vi "VI principal ( LES CHIFFRES ROMAINS).vi"() -> ()   [LabVIEW 2023]
panel:
  out "Numeric 3":dbl
  in  "ENTER AN ARAB NUMBER?":dbl
  in  "ok du roman number":bool
  out "?":string="entrez un nombre inferieur ou egale a 3000"
  out "ROMAIN NUMBER:":string
  in  "Cancel Button":bool
  in  "STOP Programme":bool
  in  "New conversion":bool
  in  "selection confirmed":bool
  in  "Enter a ROMAN  number?":string
  in  "ROMAN TO ARAB NUMBERS":string(combo) caption="WHICH CONVERSION YOU WANT?"
  in  "Arabic number":bool
  out "?":string="entrez un nombre inferieur ou egale a 3000"
  out "Arabic number:":dbl
  in  "Login":bool
  out "Login&Password":bool
  in  "Name":string
  in  "Password":string
  in  "First Name":string
  out "Message":string
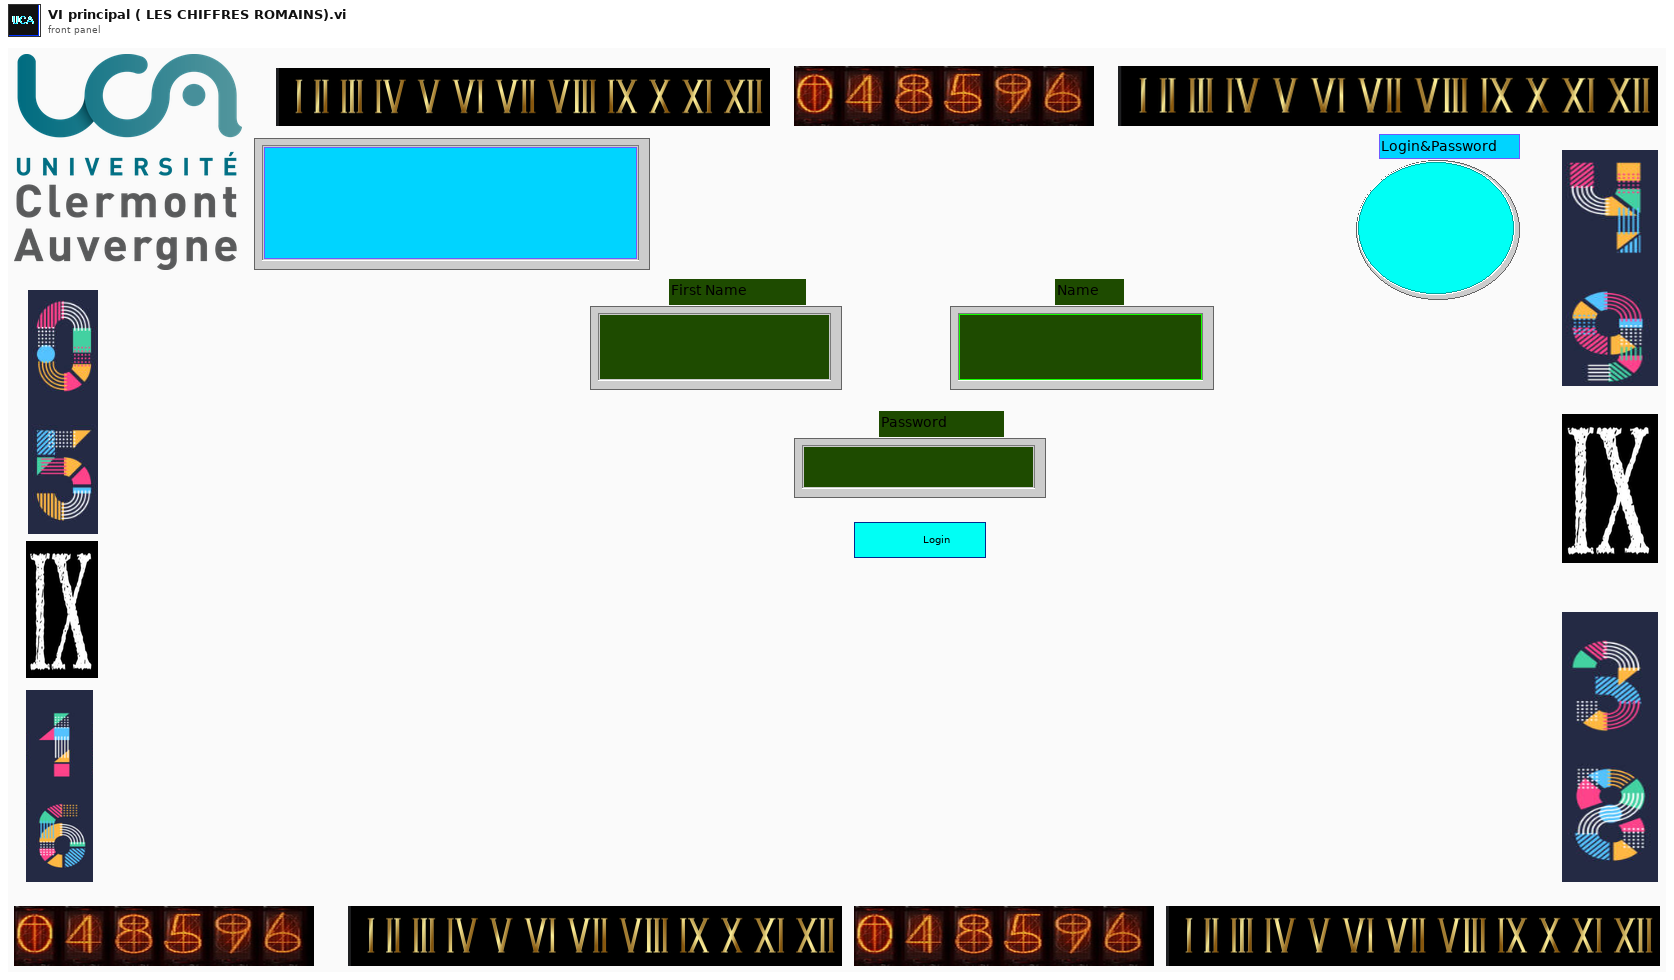
[diagram p1: front panel]
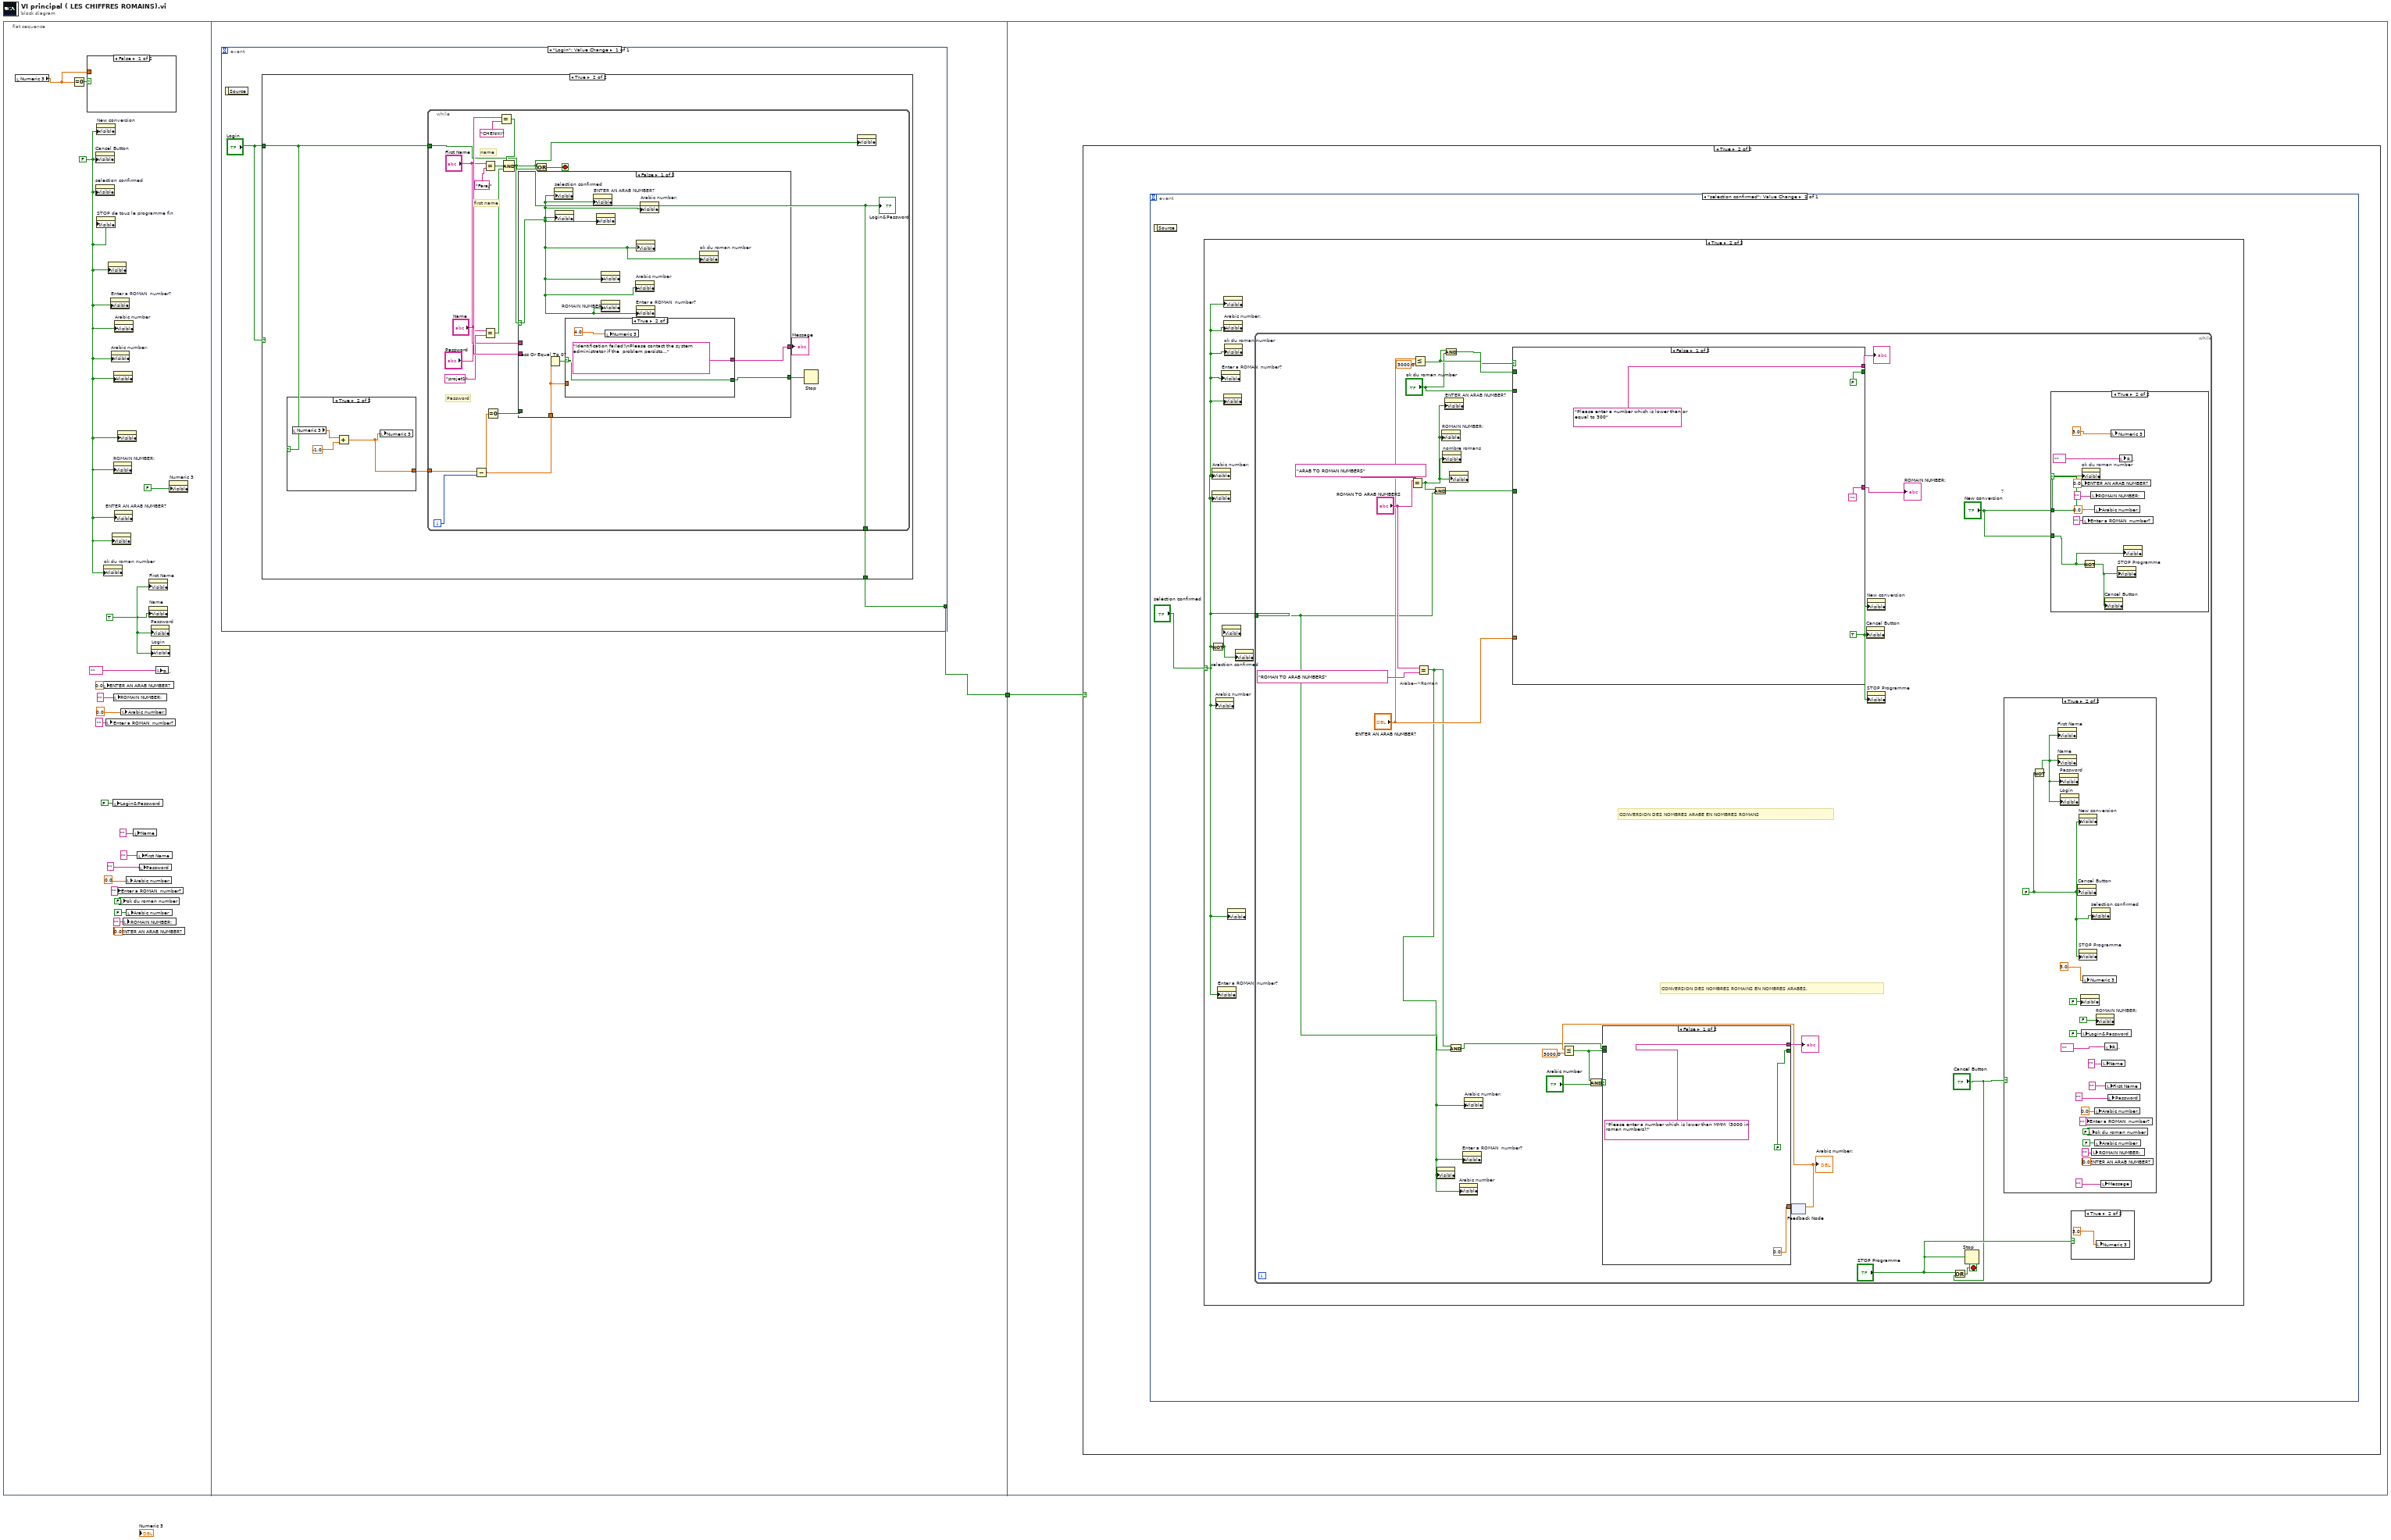
[diagram p0: block diagram]
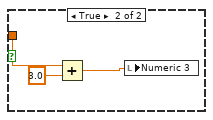
[diagram p2: hidden frame]
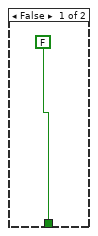
[diagram p3: hidden frame]
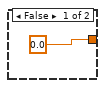
[diagram p4: hidden frame]
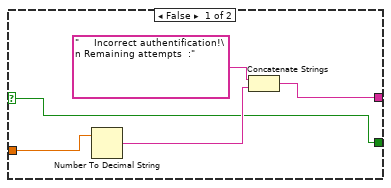
[diagram p5: hidden frame]
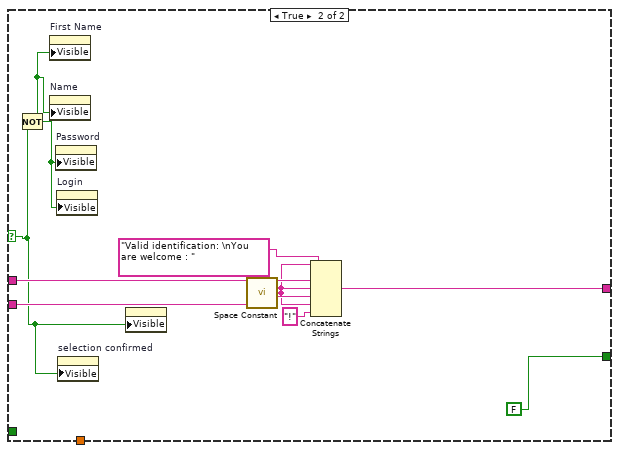
[diagram p6: hidden frame]
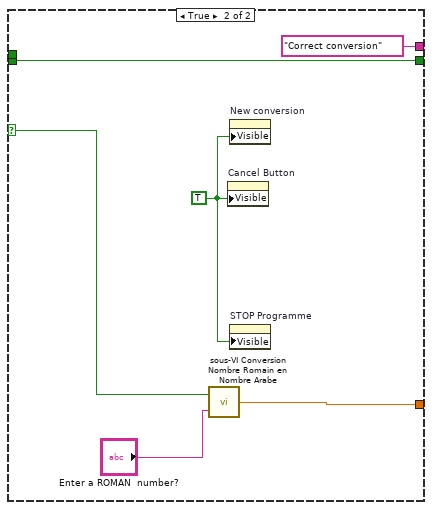
[diagram p12: hidden frame]
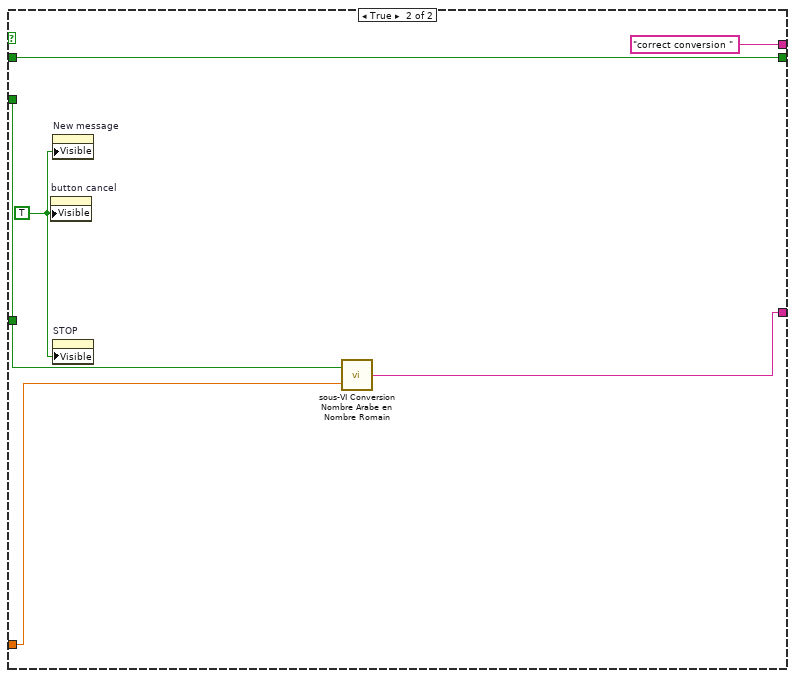
[diagram p13: hidden frame]
diagram:
  n1 = flat-sequence {
    tunnel: [w25] -> w1
    tunnel: w1 -> [w76]
    frame #0 {
      w5 = TRUE
      w21 = FALSE
      n2 = local read "Numeric 3"() -> (w2:dbl)
      n3 = Equal To 0?(x=w2) -> (x = 0?=w3:bool)
      n4 = case shown="False" w3 {
        tunnel: w2 -> [_ w24]
        frame False {
        }
        frame True {
          n5 = Add(x=w24, y=3.0) -> (x+y=w22:dbl)
          n6 = local write "Numeric 3"(w22) -> ()
        }
      }
      n7 = property on="Cancel Button" class="Bool"("Visible"=w21) -> ()  [unwired: 2 in, 2 out]
      n8 = property on="selection confirmed" class="Bool (strict)"("Visible"=w21) -> ()  [unwired: 2 in, 2 out]
      n9 = property on="New conversion" class="Bool"("Visible"=w21) -> ()  [unwired: 2 in, 2 out]
      n10 = property on="STOP de tous le programme fin" class="Bool"("Visible"=w21) -> ()  [unwired: 2 in, 2 out]
      n11 = local write "ENTER AN ARAB NUMBER?"(0.0 ("Nombre Arabe")) -> ()
      n12 = property on="ok du roman number" class="Bool (strict)"("Visible"=w21) -> ()  [unwired: 2 in, 2 out]
      n13 = local write "Enter a ROMAN  number?"("" ("Nombre romain 1")) -> ()
      n14 = property class="CmbBox"("Visible"=w21) -> ()  [unwired: 2 in, 2 out]
      n15 = property on="Enter a ROMAN  number?" class="Str"("Visible"=w21) -> ()  [unwired: 2 in, 2 out]
      n16 = property on="Arabic number:" class="DigNum (strict)"("Visible"=w21) -> ()  [unwired: 2 in, 2 out]
      n17 = property class="Str"("Visible"=w21) -> ()  [unwired: 2 in, 2 out]
      n18 = local write "Login&Password"(FALSE ("Login&Password")) -> ()
      n19 = property on="ROMAIN NUMBER:" class="Str"("Visible"=w21) -> ()  [unwired: 2 in, 2 out]
      n20 = local write "ROMAIN NUMBER:"("" ("Nombre Romain")) -> ()
      n21 = property class="CmbBox"("Visible"=w21) -> ()  [unwired: 2 in, 2 out]
      n22 = local write "Enter a ROMAN  number?"("" ("Nombre romain 1")) -> ()
      n23 = local write "ENTER AN ARAB NUMBER?"(0.0 ("Nombre Arabe")) -> ()
      n24 = property on="ENTER AN ARAB NUMBER?" class="DigNum (strict)"("Visible"=w21) -> ()  [unwired: 2 in, 2 out]
      n25 = property on="Arabic number" class="Bool (strict)"("Visible"=w21) -> ()  [unwired: 2 in, 2 out]
      n26 = property class="Str"("Visible"=w21) -> ()  [unwired: 2 in, 2 out]
      n27 = local write "ok du roman number"(FALSE ("Roman number")) -> ()
      n28 = local write "Arabic number:"(0.0 ("Nombre arabe 1")) -> ()
      n29 = local write "ROMAIN NUMBER:"("" ("Nombre Romain")) -> ()
      n30 = local write "Arabic number:"(0.0 ("Nombre arabe 1")) -> ()
      n31 = local write "Arabic number"(FALSE ("Arabic number")) -> ()
      n32 = local write "Name"("" ("First name:")) -> ()
      n33 = local write "First Name"("" ("Name:")) -> ()
      n34 = local write "Password"("" ("Password:")) -> ()
      n35 = property on="First Name" class="Str"("Visible"=w5) -> ()  [unwired: 2 in, 2 out]
      n36 = property on="Name" class="Str"("Visible"=w5) -> ()  [unwired: 2 in, 2 out]
      n37 = property on="Password" class="Str"("Visible"=w5) -> ()  [unwired: 2 in, 2 out]
      n38 = property on="Login" class="Bool (strict)"("Visible"=w5) -> ()  [unwired: 2 in, 2 out]
      n39 = local write "ROMAN TO ARAB NUMBERS"("" ("Choose your conversion")) -> ()
      n40 = property on="Numeric 3" class="DigNum (strict)"("Visible"=FALSE) -> ()  [unwired: 2 in, 2 out]
    }
    frame #1 {
      n41 = event shown="[0] \"Login\": Value Change" {
        selector: _ -> [_]
        dyn-events: _ -> [_]
        timeout: _ -> [_]
        tunnel: [w27] -> w25
        event "Login": Value Change {
          n42 = event-data() -> ()  [unwired: 1 in, 1 out]
          n43 = case shown="True" "Login" {
            tunnel: "Login" -> [_ w29]
            tunnel: [FALSE w31] -> w27
            frame False {
            }
            frame True {
              n44 = case shown="True" w29 {
                tunnel: [0.0 w33] -> w30
                frame False {
                }
                frame True {
                  n45 = local read "Numeric 3"() -> (w34:dbl)
                  n46 = Add(x=w34, y=-1.0) -> (x+y=w33:dbl)
                  n47 = local write "Numeric 3"(w33) -> ()
                }
              }
              n48 = while {
                tunnel: w29 -> [w39]
                tunnel: [w37] -> w31
                tunnel: w30 -> [w38]
                i -> [w40]
                stop <- w43 stop-if-true
                # "Password"
                # "first name"
                # "name"
                n49 = Subtract(x=w38, y=w40) -> (x-y=w41:dbl)
                n50 = Equal?(x="First Name", y="Faraj") -> (x = y?=w49:bool)
                n51 = Equal?(x="Password", y="projet1") -> (x = y?=w50:bool)
                n52 = Equal To 0?(x=w41) -> (x = 0?=w42:bool)
                n53 = Equal?(x="Name", y="CHENIKI") -> (x = y?=w48:bool)
                n54 = Compound Arithmetic op=AND(w48, w49, w50) -> (w37:bool)
                "Login&Password" <- w37
                n55 = case shown="False" w37 {
                  selector: w37 -> [w55 w68]
                  tunnel: [w57 w70] -> w53
                  tunnel: "First Name" -> [_ w74]
                  tunnel: "Name" -> [_ w73]
                  tunnel: w42 -> [_ _]
                  tunnel: w41 -> [w56 _]
                  tunnel: [w54 FALSE] -> w36
                  frame False {
                    n56 = Less Or Equal To 0?(x=w56) -> (x <= 0?=w58:bool)
                    n57 = property on="selection confirmed" class="Bool (strict)"("Visible"=w55) -> ()  [unwired: 2 in, 2 out]
                    n58 = property class="CmbBox"("Visible"=w55) -> ()  [unwired: 2 in, 2 out]
                    n59 = case shown="True" w58 {
                      selector: w58 -> [w59 w64]
                      tunnel: [w62 "Identification failed!\nPlease contact the system administrator if the  problem persists..." ("string")] -> w57
                      tunnel: w56 -> [w61 _]
                      tunnel: [w59 w64] -> w54
                      frame False {
                        n60 = Number To Decimal String(number=w61) -> (decimal integer string=w60:string)  [unwired: 1 in]
                        n61 = Concatenate Strings("     Incorrect authentification!\n Remaining attempts  :", w60) -> (w62:string)
                      }
                      frame True {
                        n62 = local write "Numeric 3"(4.0) -> ()
                      }
                    }
                    n63 = property on="ENTER AN ARAB NUMBER?" class="DigNum (strict)"("Visible"=w55) -> ()  [unwired: 2 in, 2 out]
                    n64 = property class="Str"("Visible"=w55) -> ()  [unwired: 2 in, 2 out]
                    n65 = property class="Str"("Visible"=w55) -> ()  [unwired: 2 in, 2 out]
                    n66 = property on="ROMAIN NUMBER:" class="Str"("Visible"=w55) -> ()  [unwired: 2 in, 2 out]
                    n67 = property on="Arabic number" class="Bool (strict)"("Visible"=w55) -> ()  [unwired: 2 in, 2 out]
                    n68 = property on="Enter a ROMAN  number?" class="Str"("Visible"=w55) -> ()  [unwired: 2 in, 2 out]
                    n69 = property class="Str"("Visible"=w55) -> ()  [unwired: 2 in, 2 out]
                    n70 = property on="Arabic number:" class="DigNum (strict)"("Visible"=w55) -> ()  [unwired: 2 in, 2 out]
                    n71 = property on="ok du roman number" class="Bool (strict)"("Visible"=w55) -> ()  [unwired: 2 in, 2 out]
                  }
                  frame True {
                    n72 = Not(x=w68) -> (.not. x?=w69:bool)
                    n73 = property on="First Name" class="Str"("Visible"=w69) -> ()  [unwired: 2 in, 2 out]
                    n74 = property on="Name" class="Str"("Visible"=w69) -> ()  [unwired: 2 in, 2 out]
                    n75 = property on="Password" class="Str"("Visible"=w69) -> ()  [unwired: 2 in, 2 out]
                    n76 = property on="Login" class="Bool (strict)"("Visible"=w69) -> ()  [unwired: 2 in, 2 out]
                    n77 = property on="selection confirmed" class="Bool (strict)"("Visible"=w68) -> ()  [unwired: 2 in, 2 out]
                    n78 = property class="CmbBox"("Visible"=w68) -> ()  [unwired: 2 in, 2 out]
                    n79 = call <vilib>:"Space Constant.vi"() -> ("String"=w72:string)
                    n80 = Concatenate Strings("Valid identification: \nYou are welcome : ", w72, w74, w72, w73, w72, "!") -> (w70:string)
                  }
                }
                "Message" <- w53
                n81 = Or(x=w37, y=w39) -> (x .or. y?=w43:bool)
                n82 = Stop(stop? (T)=w36) -> ()
                n83 = property class="CmbBox"("Visible"=w37) -> ()  [unwired: 2 in, 2 out]
              }
            }
          }
        }
      }
    }
    frame #2 {
      n84 = case shown="True" w76 {
        frame False {
        }
        frame True {
          n85 = event shown="[0] \"selection confirmed\": Value Change" {
            selector: _ -> [_]
            dyn-events: _ -> [_]
            timeout: _ -> [_]
            event "selection confirmed": Value Change {
              n86 = event-data() -> ()  [unwired: 1 in, 1 out]
              n87 = case shown="True" "selection confirmed" {
                selector: "selection confirmed" -> [_ w79]
                frame False {
                }
                frame True {
                  n88 = Not(x=w79) -> (.not. x?=w78:bool)
                  n89 = property on="Arabic number:" class="DigNum (strict)"("Visible"=w79) -> ()  [unwired: 2 in, 2 out]
                  n90 = property class="Str"("Visible"=w79) -> ()  [unwired: 2 in, 2 out]
                  n91 = property on="Arabic number" class="Bool (strict)"("Visible"=w79) -> ()  [unwired: 2 in, 2 out]
                  n92 = property on="Enter a ROMAN  number?" class="Str"("Visible"=w79) -> ()  [unwired: 2 in, 2 out]
                  n93 = property on="Enter a ROMAN  number?" class="Str"("Visible"=w79) -> ()  [unwired: 2 in, 2 out]
                  n94 = property class="CmbBox"("Visible"=w78) -> ()  [unwired: 2 in, 2 out]
                  n95 = property class="Str"("Visible"=w79) -> ()  [unwired: 2 in, 2 out]
                  n96 = property class="CmbBox"("Visible"=w79) -> ()  [unwired: 2 in, 2 out]
                  n97 = property on="Arabic number:" class="DigNum (strict)"("Visible"=w79) -> ()  [unwired: 2 in, 2 out]
                  n98 = property on="ok du roman number" class="Bool (strict)"("Visible"=w79) -> ()  [unwired: 2 in, 2 out]
                  n99 = property class="Str"("Visible"=w79) -> ()  [unwired: 2 in, 2 out]
                  n100 = property on="selection confirmed" class="Bool (strict)"("Visible"=w78) -> ()  [unwired: 2 in, 2 out]
                  n101 = while {
                    tunnel: w79 -> [w91]
                    stop <- w87 stop-if-true
                    w90 = TRUE
                    # "CONVERSION DES NOMBRES ARABE EN NOMBRES ROMANS"
                    # "CONVERSION DES NOMBRES ROMAINS EN NOMBRES ARABES."
                    # "?"
                    # "Arabe-->Roman"
                    n102 = Equal?(x="ROMAN TO ARAB NUMBERS", y="ARAB TO ROMAN NUMBERS") -> (x = y?=w96:bool)
                    n103 = Less Or Equal?(x="ENTER AN ARAB NUMBER?", y=3000.0) -> (x <= y?=w100:bool)
                    n104 = Equal?(x="ROMAN TO ARAB NUMBERS", y="ROMAN TO ARAB NUMBERS") -> (x = y?=w80:bool)
                    n105 = And(x=w96, y=w91) -> (x .and. y?=w97:bool)
                    n106 = property class="Str"("Visible"=w80) -> ()  [unwired: 2 in, 2 out]
                    n107 = property on="ROMAIN NUMBER:" class="Str"("Visible"=w96) -> ()  [unwired: 2 in, 2 out]
                    n108 = property on="nombre romans" class="Bool (strict)"("Visible"=w96) -> ()  [unwired: 2 in, 2 out]
                    n109 = And(x=w100, y="ok du roman number") -> (x .and. y?=w98:bool)
                    n110 = property on="ENTER AN ARAB NUMBER?" class="DigNum (strict)"("Visible"=w96) -> ()  [unwired: 2 in, 2 out]
                    n111 = And(x=w80, y=w91) -> (x .and. y?=w81:bool)
                    n112 = property class="Str"("Visible"=w96) -> ()  [unwired: 2 in, 2 out]
                    n113 = property on="Arabic number" class="Bool (strict)"("Visible"=w80) -> ()  [unwired: 2 in, 2 out]
                    n114 = property on="Enter a ROMAN  number?" class="Str"("Visible"=w80) -> ()  [unwired: 2 in, 2 out]
                    n115 = property on="Arabic number:" class="DigNum (strict)"("Visible"=w80) -> ()  [unwired: 2 in, 2 out]
                    n116 = case shown="False" w98 {
                      tunnel: "ENTER AN ARAB NUMBER?" -> [_ w148]
                      tunnel: ["Please enter a number which is lower than or equal to 300" "correct conversion "] -> w101
                      tunnel: w100 -> [_ w151]
                      tunnel: [FALSE w151] -> _
                      tunnel: ["" w147] -> w99
                      tunnel: w97 -> [_ _]
                      tunnel: "ok du roman number" -> [_ w146]
                      frame False {
                      }
                      frame True {
                        w149 = TRUE
                        n117 = property on="button cancel" class="Bool"("Visible"=w149) -> ()  [unwired: 2 in, 2 out]
                        n118 = property on="New message" class="Bool"("Visible"=w149) -> ()  [unwired: 2 in, 2 out]
                        n119 = property on="STOP" class="Bool"("Visible"=w149) -> ()  [unwired: 2 in, 2 out]
                        n120 = call "sous-VI Conversion Nombre Arabe en Nombre Romain.vi"("Enter AN ARABIC NUMBER?"=w148, "Roman number"=w146) -> ("ROMAN NUMBER:"=w147:string)
                      }
                    }
                    "?" <- w101
                    "ROMAIN NUMBER:" <- w99
                    n121 = feedback #1() -> (w85:dbl)  [unwired: 1 in]
                    "Arabic number:" <- w85
                    n122 = Less Or Equal?(x=w85, y=3000.0) -> (x <= y?=w95:bool)
                    n123 = And(x=w95, y="Arabic number") -> (x .and. y?=w92:bool)
                    n124 = case shown="False" w92 {
                      selector: w92 -> [_ w138]
                      tunnel: ["Please enter a number which is lower than MMM  (3000 in roman numbers)!" "Correct conversion"] -> w94
                      tunnel: [FALSE w141] -> _
                      tunnel: w95 -> [_ w141]
                      tunnel: [0.0 w139] -> w86
                      tunnel: w81 -> [_ _]
                      frame False {
                      }
                      frame True {
                        w140 = TRUE
                        n125 = call "sous-VI Conversion Nombre Romain en Nombre Arabe.vi"("Enter a ROMAN nomber?"="Enter a ROMAN  number?", "RESULT"=w138) -> ("Arabic number:"=w139:dbl)
                        n126 = property on="Cancel Button" class="Bool"("Visible"=w140) -> ()  [unwired: 2 in, 2 out]
                        n127 = property on="New conversion" class="Bool"("Visible"=w140) -> ()  [unwired: 2 in, 2 out]
                        n128 = property on="STOP Programme" class="Bool"("Visible"=w140) -> ()  [unwired: 2 in, 2 out]
                      }
                    }
                    "?" <- w94
                    n129 = feedback-in #1(w86) -> ()
                    n130 = property on="Cancel Button" class="Bool"("Visible"=w90) -> ()  [unwired: 2 in, 2 out]
                    n131 = property on="New conversion" class="Bool"("Visible"=w90) -> ()  [unwired: 2 in, 2 out]
                    n132 = property on="STOP Programme" class="Bool"("Visible"=w90) -> ()  [unwired: 2 in, 2 out]
                    n133 = Or(x="STOP Programme", y="Cancel Button") -> (x .or. y?=w87:bool)
                    n134 = Stop(stop? (T)="STOP Programme") -> ()
                    n135 = case shown="True" "Cancel Button" {
                      frame False {
                      }
                      frame True {
                        w117 = FALSE
                        n136 = Not(x=w117) -> (.not. x?=w118:bool)
                        n137 = property on="First Name" class="Str"("Visible"=w118) -> ()  [unwired: 2 in, 2 out]
                        n138 = property on="Name" class="Str"("Visible"=w118) -> ()  [unwired: 2 in, 2 out]
                        n139 = property on="Password" class="Str"("Visible"=w118) -> ()  [unwired: 2 in, 2 out]
                        n140 = property on="Login" class="Bool (strict)"("Visible"=w118) -> ()  [unwired: 2 in, 2 out]
                        n141 = property on="Cancel Button" class="Bool"("Visible"=w117) -> ()  [unwired: 2 in, 2 out]
                        n142 = property on="New conversion" class="Bool"("Visible"=w117) -> ()  [unwired: 2 in, 2 out]
                        n143 = property on="STOP Programme" class="Bool"("Visible"=w117) -> ()  [unwired: 2 in, 2 out]
                        n144 = property class="CmbBox"("Visible"=FALSE) -> ()  [unwired: 2 in, 2 out]
                        n145 = local write "Login&Password"(FALSE ("Login&Password")) -> ()
                        n146 = local write "Enter a ROMAN  number?"("" ("Nombre romain 1")) -> ()
                        n147 = local write "ENTER AN ARAB NUMBER?"(0.0 ("Nombre Arabe")) -> ()
                        n148 = local write "Numeric 3"(3.0) -> ()
                        n149 = local write "ok du roman number"(FALSE ("Roman number")) -> ()
                        n150 = property on="selection confirmed" class="Bool (strict)"("Visible"=w117) -> ()  [unwired: 2 in, 2 out]
                        n151 = local write "ROMAIN NUMBER:"("" ("Nombre Romain")) -> ()
                        n152 = local write "Arabic number:"(0.0 ("Nombre arabe 1")) -> ()
                        n153 = local write "Arabic number"(FALSE ("Arabic number")) -> ()
                        n154 = property on="ROMAIN NUMBER:" class="Str"("Visible"=FALSE) -> ()  [unwired: 2 in, 2 out]
                        n155 = local write "Message"("" ("String")) -> ()
                        n156 = local write "Name"("" ("First name:")) -> ()
                        n157 = local write "ROMAN TO ARAB NUMBERS"("" ("Choose your conversion")) -> ()
                        n158 = local write "First Name"("" ("Name:")) -> ()
                        n159 = local write "Password"("" ("Password:")) -> ()
                      }
                    }
                    n160 = case shown="True" "New conversion" {
                      tunnel: "New conversion" -> [_ w108]
                      tunnel: "New conversion" -> [_ w109]
                      frame False {
                        # "?"
                      }
                      frame True {
                        n161 = local write "ENTER AN ARAB NUMBER?"(0.0 ("Nombre Arabe")) -> ()
                        n162 = property on="ok du roman number" class="Bool (strict)"("Visible"=w109) -> ()  [unwired: 2 in, 2 out]
                        n163 = Not(x=w108) -> (.not. x?=w110:bool)
                        n164 = local write "Enter a ROMAN  number?"("" ("Nombre romain 1")) -> ()
                        n165 = local write "ROMAIN NUMBER:"("" ("Nombre Romain")) -> ()
                        n166 = local write "Arabic number:"(0.0 ("Nombre arabe 1")) -> ()
                        n167 = property on="Cancel Button" class="Bool"("Visible"=w110) -> ()  [unwired: 2 in, 2 out]
                        n168 = local write "Numeric 3"(3.0) -> ()
                        n169 = property on="STOP Programme" class="Bool"("Visible"=w110) -> ()  [unwired: 2 in, 2 out]
                        n170 = local write "ROMAN TO ARAB NUMBERS"("" ("Choose your conversion")) -> ()
                        n171 = property class="CmbBox"("Visible"=w108) -> ()  [unwired: 2 in, 2 out]
                      }
                    }
                    n172 = case shown="True" "STOP Programme" {
                      frame False {
                      }
                      frame True {
                        n173 = local write "Numeric 3"(3.0) -> ()
                      }
                    }
                  }
                }
              }
            }
          }
        }
      }
    }
  }
